vi "SetTest.vi"(8 "error in (no error)":errorcluster, 10 "Test":T1={"Code"="", "Name"="", "Description"="", "Group"="", "IsGroup"=FALSE, "Tag"="", "Method"="", "Parrameter"="", "DataType"=enum."String", "Value"=variant, "Status"=enum."Pass", "LimitLo"=variant, "LimitHi"=variant, "StringMatch"="", "BooleanMatch"=FALSE, "DisplayFormat"="", "Units"="", "TestTime"=0.0}, 11 "reference in":refnum<class "TestView_Tree_Single.lvclass">) -> (0 "error out":errorcluster, 3 "reference in":refnum<class "TestView_Tree_Single.lvclass">)   [LabVIEW 2022 SP3, in "TestView_Tree_Single.lvlib" / "TestView_Tree_Single.lvclass"]
uses:
  TestView_Tree_Single.lvclass
  Components/MES_Base.lvlibp/Controls/Test.ctl
  Components/MES_Base.lvlibp/MES_Base.lvclass
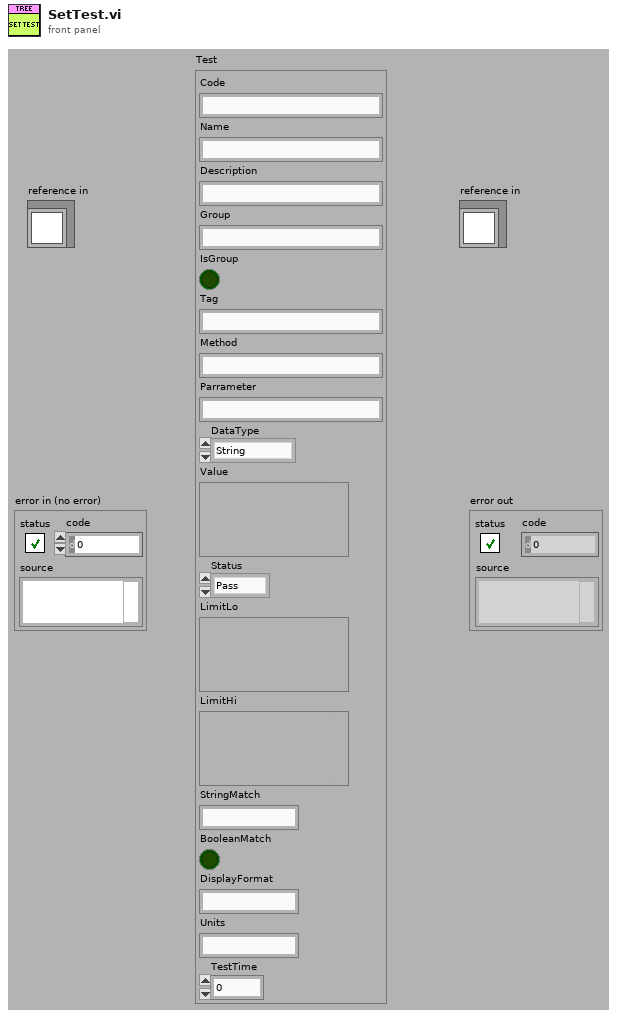
[diagram p1: front panel]
types:
  T1 = typedef "MES_Base.lvlibp/MES_Base.lvclass/Test.ctl" = cluster{"Code":string, "Name":string, "Description":string, "Group":string, "IsGroup":bool, "Tag":string, "Method":string, "Parrameter":string, "DataType":enum16{"NA", "String", "Boolean", "Int", "Dbl"}, "Value":variant, "Status":enum16{"Pending", "Pass", "Fail"}, "LimitLo":variant, "LimitHi":variant, "StringMatch":string, "BooleanMatch":bool, "DisplayFormat":string, "Units":string, "TestTime":dbl}
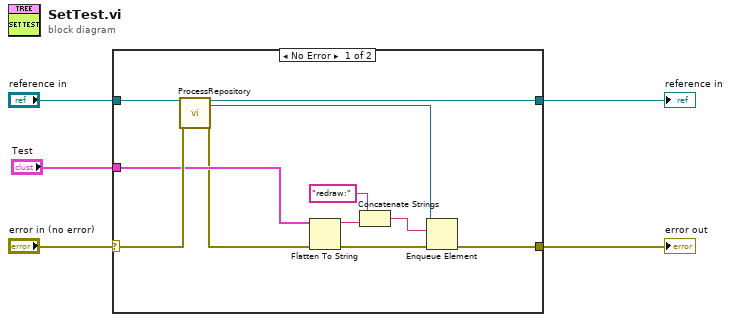
[diagram p0: block diagram]
diagram:
  n1 = case shown="No Error" "error in (no error)" {
    selector: "error in (no error)" -> [w10 w17]
    tunnel: "reference in" -> [w12 w18]
    tunnel: "Test" -> [w8 _]
    tunnel: [w6 w17] -> w3
    tunnel: [w11 w18] -> w2
    frame No Error {
      n2 = call "ProcessRepository.vi"("reference in"=w12, "error in (no error)"=w10) -> ("reference out"=w11:refnum<class "TestView_Tree_Single.lvclass">, "ToProcessQueue"=w9:refnum<queue>, "error out"=w7:errorcluster)  [unwired: 11 in, 4 out]
      n3 = Flatten To String(anything=w8, error in (no error)=w7) -> (data string=w15:string, error out=w14:errorcluster)  [unwired: 2 in, 1 out]
      n4 = Concatenate Strings("redraw:" ("string"), w15) -> (w16:string)
      n5 = Enqueue Element(queue=w9, element=w16, error in (no error)=w14) -> (error out=w6:errorcluster)  [unwired: 1 in, 2 out]
    }
    frame Error {
    }
  }
  "error out" <- w3
  "reference in" <- w2
